vi "TDT-AODO-Initialize.vi"(0 "RPcox":refnum<k7>, 7 "Config":T1, 11 "error in (no error)":errorcluster) -> (15 "error out":errorcluster)   [LabVIEW 2020]
uses:
  Typedefs/TDT-AODO-Config.ctl
  Typedefs/TDT-AODO-Output Spec.ctl
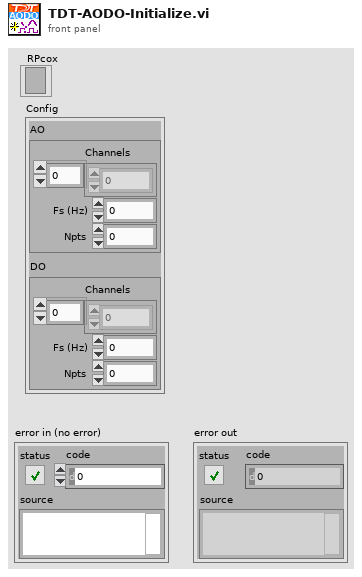
[diagram p1: front panel]
types:
  T1 = typedef "TDT-AODO-Config.ctl" = cluster{"AO":T2, "DO":T2}
  T2 = typedef "TDT-AODO-Output Spec.ctl" = cluster{"Channels":i32[], "Fs (Hz)":dbl, "Npts":i32}
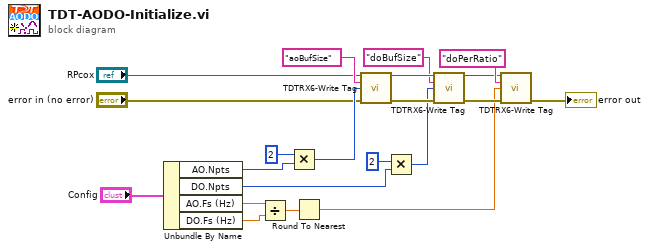
[diagram p0: block diagram]
diagram:
  n1 = Unbundle By Name("Config") -> ("AO.Npts"=w8:i32, "DO.Npts"=w7:i32, "AO.Fs (Hz)"=w6:dbl, "DO.Fs (Hz)"=w5:dbl)
  n2 = Divide(x=w6, y=w5) -> (x/y=w4:dbl)
  n3 = Multiply(x=2, y=w8) -> (x*y=w16:i32)
  n4 = Round To Nearest(number=w4) -> (nearest integer value=w3:dbl)
  n5 = call "TDTRX6-Write Tag.vi"("RPcox"="RPcox", "Name"="aoBufSize", "Value"=w16, "error in"="error in (no error)") -> ("RPcox Out"=w19:refnum<k7>, "error out"=w20:errorcluster)  [unwired: 10 in]
  n6 = Multiply(x=2, y=w7) -> (x*y=w11:i32)
  n7 = call "TDTRX6-Write Tag.vi"("RPcox"=w19, "Name"="doBufSize", "Value"=w11, "error in"=w20) -> ("RPcox Out"=w14:refnum<k7>, "error out"=w13:errorcluster)  [unwired: 10 in]
  n8 = call "TDTRX6-Write Tag.vi"("RPcox"=w14, "Name"="doPerRatio", "Value"=w3, "error in"=w13) -> ("error out"=→"error out":errorcluster)  [unwired: 10 in, 1 out]
